vi "Autonomous.vi"   [LabVIEW 2018]
doc: "This VI starts when autonomous period begins, and will automatically be terminated when it ends. You can carry out timed or sensor driven operations directly to I/O or to subsystems without needing to return to the caller."
uses:
  <vilib>/Rock Robotics/Network Tables/NT Read String.vi
  Auton/Auton Kill Switch.vi
types:
  T1 = typedef "WPI_DriverStationMatch Info.ctl" = cluster{"Autonomous Elapsed Seconds":dbl, "TeleOp Elapsed Seconds":dbl, "Disabled Elapsed Seconds":dbl, "Visited Autonomous":bool, "Visited TeleOp":bool, "Visited Disabled":bool, "Autonomous Settings":cluster{"Autonomous Style":enum16{"Iterative", "Independent"}, "VI Refnum":refnum<vi>}}
  T2 = typedef "WPI_DriverStationDerivedRobotMode.ctl" = enum16{"Init", "Execute", "Stop"}
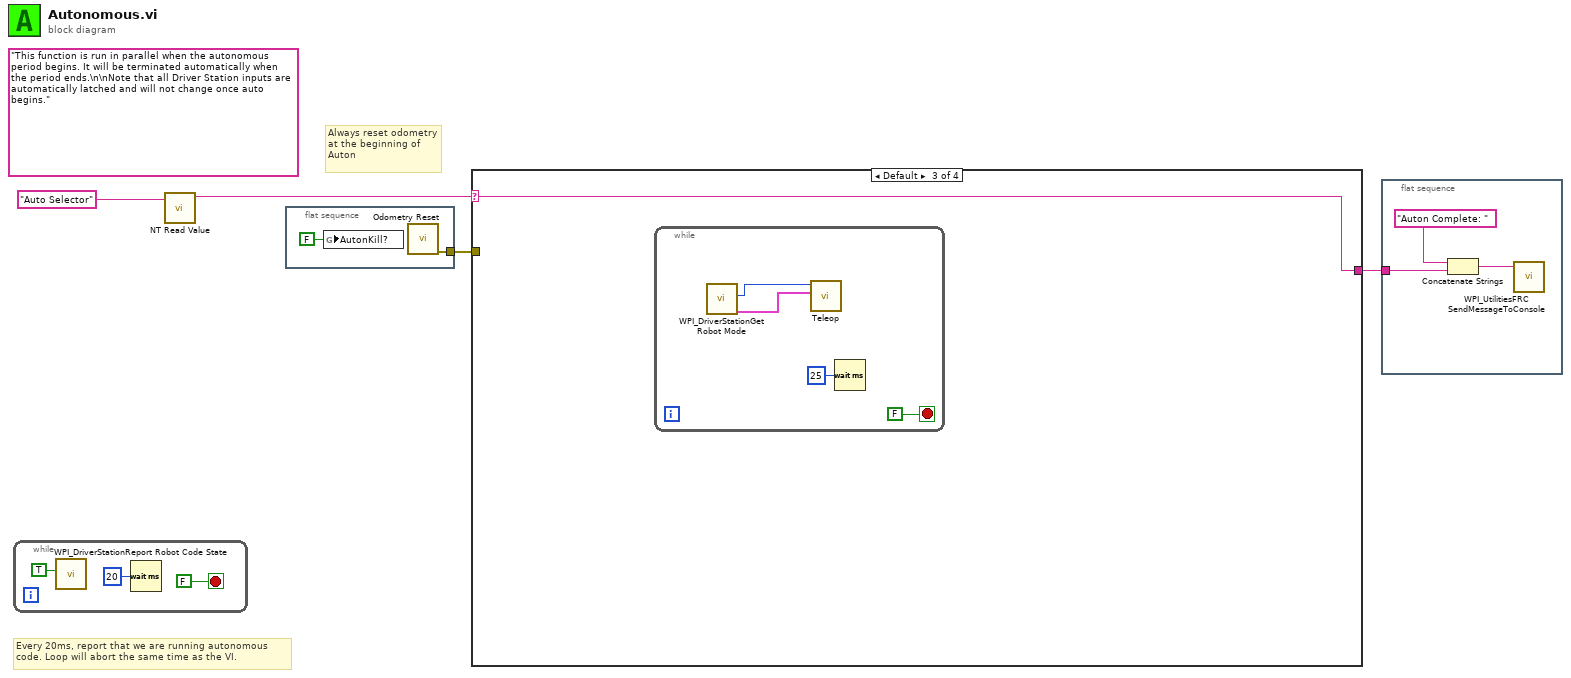
[diagram p0: block diagram]
diagram:
  (unwired) "This function is run in parallel when the autonomous period begins. It will be terminated automatically when the period ends.\n\nNote that all Driver Station inputs are automatically latched and will not change once auto begins."
  # "Always reset odometry at the beginning of Auton"
  # "Every 20ms, report that we are running autonomous\ncode. Loop will abort the same time as the VI."
  n1 = while {
    stop <- FALSE stop-if-true
    n2 = call <vilib>:"WPI_DriverStationReport Robot Code State.vi"("Autonomous"=TRUE) -> ()  [unwired: 10 in, 1 out]
    n3 = Wait (ms)(milliseconds to wait=u32 20) -> ()  [unwired: 1 out]
  }
  n4 = call-poly <vilib>:"NT Read Value.vi"("Name"="Auto Selector") -> ("String"=w1:string)  [unwired: 9 in, 1 out]
  n5 = flat-sequence {
    tunnel: [w9] -> w3
    frame #0 {
      n6 = global write "Auton Kill Switch.vi" "AutonKill?"(FALSE ("AutonKill?")) -> ()
      n7 = call "Odometry Reset.vi"() -> ("error out"=w9:errorcluster)  [unwired: 11 in]
    }
  }
  n8 = case shown="Default" w1 {
    selector: w1 -> [w10 w11 w12 w17]
    tunnel: w3 -> [_ _ _ _]
    tunnel: [w10 w11 w12 w17] -> w2
    frame "Alternative 1" {
    }
    frame "Backup NT Auton" {
    }
    frame Default {
      n9 = while {
        stop <- FALSE stop-if-true
        n10 = call <vilib>:"WPI_DriverStationGet Robot Mode.vi"() -> ("Match Info out"=w13:T1, "Call Context"=w14:T2)  [unwired: 2 in, 8 out]
        n11 = call "Teleop.vi"("Match Info"=w13, "Call Context"=w14) -> ()  [unwired: 10 in]
        n12 = Wait (ms)(milliseconds to wait=u32 25) -> ()  [unwired: 1 out]
      }
    }
    frame "Alternative 2" {
    }
  }
  n13 = flat-sequence {
    tunnel: w2 -> [w18]
    frame #0 {
      n14 = Concatenate Strings("Auton Complete: " ("Message"), w18) -> (w19:string)
      n15 = call <vilib>:"WPI_UtilitiesFRC SendMessageToConsole.vi"("Message"=w19) -> ()  [unwired: 14 in, 1 out]
    }
  }
